vi "host.vi"() -> ()   [LabVIEW 2010]
uses:
  <vilib>/userDefined/High Color/nirio_resource_hc.ctl
  <vilib>/rvi/interface/nirviOpenFPGA/nirviOpenFPGA.xnode
  FPGA Bitfiles/FPGATarget2_main.lvbitx
  main.vi
  <vilib>/rvi/ClientSDK/nirviWhatTheDeviceIsDoing.ctl
  <vilib>/rvi/interface/nirviMethod/nirviMethod.xnode
  <vilib>/rvi/interface/nirviReadWriteControl/nirviReadWriteControl.xnode
  <vilib>/rvi/interface/common/niFpgaNodeNameForErrorReporting.ctl
  <vilib>/rvi/errors/niLvFpgaWhatHappensToTopLevelVI.ctl
  <vilib>/rvi/interface/nirviCloseFPGA/nirviCloseFPGA.xnode
  <vilib>/Utility/file.llb/Write To Spreadsheet File (I64).vi
  <vilib>/FPGAPlugInAG/PXI-7813R/niLvFpga_Open_PXI-7813R.vi
  <vilib>/FPGAPlugInAG/PXI-7813R/niLvFpga_Reset_PXI-7813R.vi
  <vilib>/Utility/error.llb/Error Cluster From Error Code.vi
  <vilib>/rvi/errors/niLvFpgaAdjustHostInterfaceError.vi
  <vilib>/FPGAPlugInAG/PXI-7813R/niLvFpga_Close_PXI-7813R.vi
  NiFpgaLv.dll
panel:
  in  "file path (dialog if empty)":path
  out "Timed Out?":bool
  in  "Number of Elements":u32=65000
  out "Elements Remaining":u32
  out "Waveform Graph":u16[](graph)
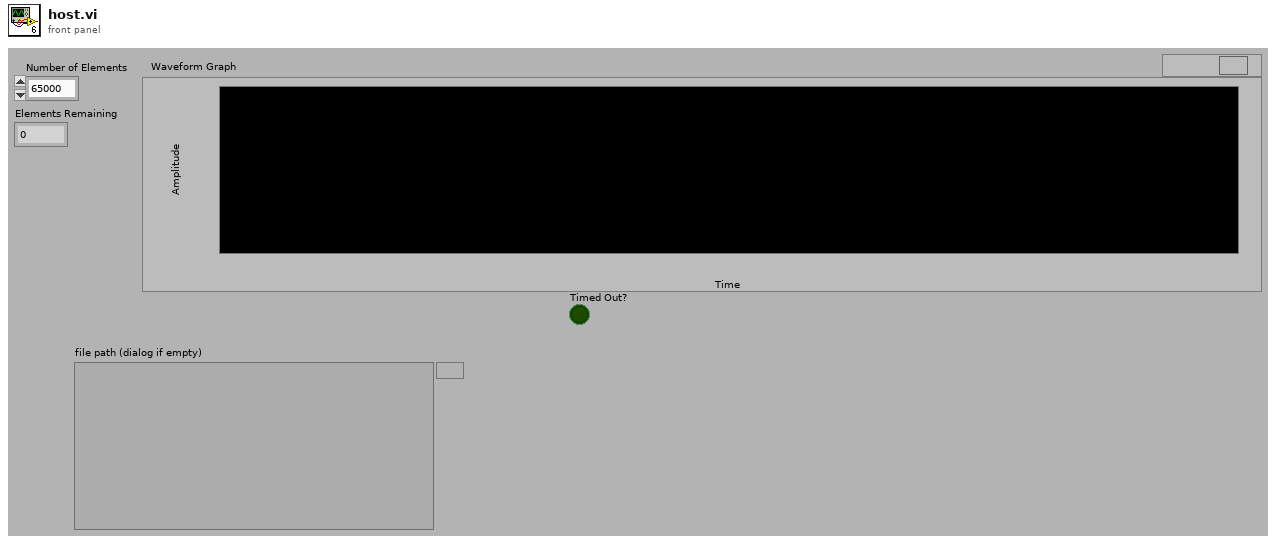
[diagram p1: front panel]
types:
  T1 = typedef "nirio_resource_hc.ctl" = tag
  T2 = typedef "niFpgaNodeNameForErrorReporting.ctl" = enum16{"Open FPGA VI Reference", "Read/Write Control", "Invoke Method: Abort", "Invoke Method: Acknowledge IRQ", "Invoke Method: Download", "Invoke Method: FIFO.Configure", "Invoke Method: FIFO.Read", "Invoke Method: FIFO.Start", "Invoke Method: FIFO.Stop", "Invoke Method: FIFO.Write", "Invoke Method: Reset", "Invoke Method: Run", "Invoke Method: Wait on IRQ", "Close FPGA VI Reference"}
  T3 = typedef "niLvFpgaWhatHappensToTopLevelVI.ctl" = enum16{"top level VI scripted behind XNode", "top level VI inlined behind XNode"}
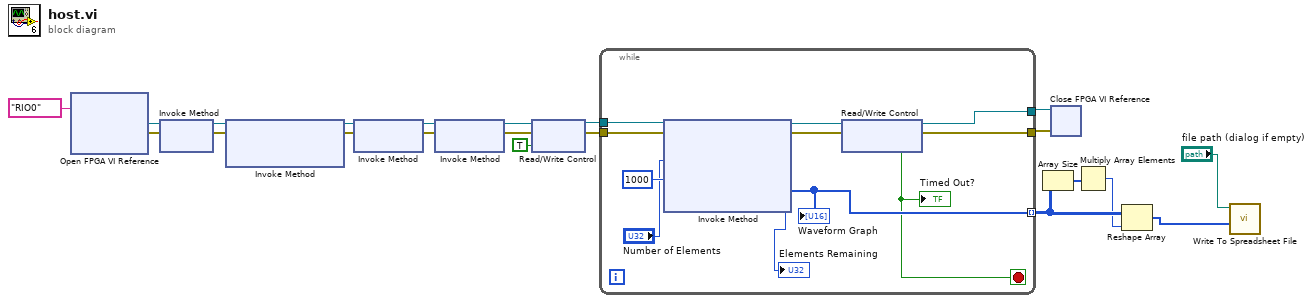
[diagram p0: block diagram]
diagram:
  n1 = xnode "Open FPGA VI Reference"("resource name"=T1 "RIO0") -> ("FPGA VI Reference Out"=w9:refnum<k20>, "error out"=w14:errorcluster)  [unwired: 1 in]
  n2 = xnode "Invoke Method"("FPGA VI Reference In"=w9, "error in"=w14) -> ("FPGA VI Reference Out"=w12:refnum<k20>, "error out"=w13:errorcluster)
  n3 = xnode "Invoke Method"("FPGA VI Reference In"=w12, "error in"=w13) -> ("FPGA VI Reference Out"=w1:refnum<k20>, "error out"=w8:errorcluster)  [unwired: 1 in]
  n4 = xnode "Invoke Method"("FPGA VI Reference In"=w1, "error in"=w8) -> ("FPGA VI Reference Out"=w10:refnum<k20>, "error out"=w11:errorcluster)
  n5 = xnode "Invoke Method"("FPGA VI Reference In"=w10, "error in"=w11) -> ("FPGA VI Reference Out"=w7:refnum<k20>, "error out"=w5:errorcluster)
  n6 = xnode "Read/Write Control"("FPGA VI Reference In"=w7, "error in"=w5, "start"=TRUE) -> ("FPGA VI Reference Out"=w6:refnum<k20>, "error out"=w4:errorcluster)
  n7 = while {
    tunnel: w6 -> [w32]
    tunnel: w4 -> [w31]
    tunnel: [w26] -> w20
    tunnel: [w24] -> w19
    tunnel: [w23] -> w17 mode=indexing
    stop <- w22 stop-if-true
    n8 = xnode "Invoke Method"("FPGA VI Reference In"=w32, "error in"=w31, "Number of Elements"="Number of Elements", "Timeout (ms)"=1000) -> ("FPGA VI Reference Out"=w25:refnum<k20>, "error out"=w27:errorcluster, "Data"=w23:u16[], "Elements Remaining"=→"Elements Remaining":u32)
    "Waveform Graph" <- w23
    n9 = xnode "Read/Write Control"("FPGA VI Reference In"=w25, "error in"=w27) -> ("FPGA VI Reference Out"=w24:refnum<k20>, "error out"=w26:errorcluster, "Timed Out?"=w22:bool)
    "Timed Out?" <- w22
  }
  n10 = Array Size(array=w17) -> (size(s)=w16:i32[])
  n11 = xnode "Close FPGA VI Reference"("FPGA VI Reference In"=w19, "error in"=w20) -> ()  [unwired: 1 out]
  n12 = Multiply Array Elements(1:w16) -> (0:w15:i32)
  n13 = Reshape Array(w17, w15) -> (w18:u16[])
  n14 = call-poly <vilib>:"Write To Spreadsheet File.vi"("1D data"=w18, "file path (dialog if empty)"="file path (dialog if empty)") -> ()  [unwired: 6 in, 1 out]
